vi "format_string_activity23.vi"() -> ()   [LabVIEW 2025]
panel:
  out "Length of string":i32
  out "Combined string":string
  in  "Trailer":string
  in  "Number":dbl
  in  "Header":string
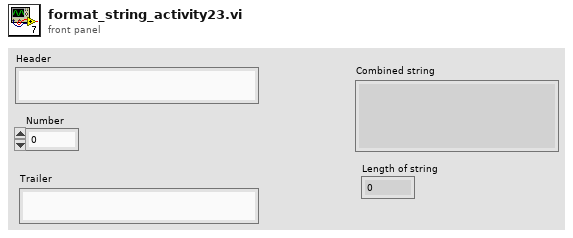
[diagram p1: front panel]
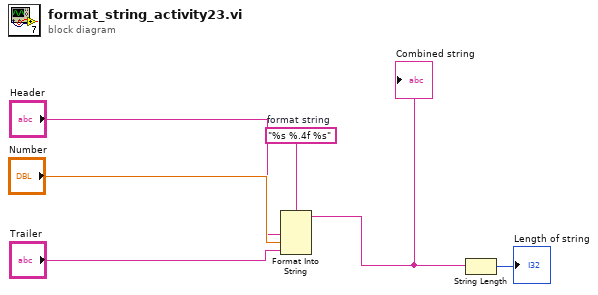
[diagram p0: block diagram]
diagram:
  w5 = "%s %.4f %s"  # format string
  n1 = Format Into String(format string=w5, "Header", "Number", "Trailer") -> (resulting string=w3:string)  [unwired: 2 in, 1 out]
  "Combined string" <- w3
  n2 = String Length(string=w3) -> (length=→"Length of string":i32)
